vi "Close.vi"(8 "error in":errorcluster, 11 "OnOff in":refnum<class "OnOff.lvclass">) -> (0 "error out":errorcluster, 3 "OnOff out":refnum<class "OnOff.lvclass">)   [LabVIEW 2023, in "OnOff.lvclass"]
uses:
  OnOff.lvclass
  OnOff.lvclass/OnOff.ctl
  <vilib>/ADAS Replay HIL/AdasHilServices/AdasHilServices Fill In Error Info Ex.vi
  <vilib>/ADAS Replay HIL/AdasHilServices/AdasHilChannelServices.lvlib
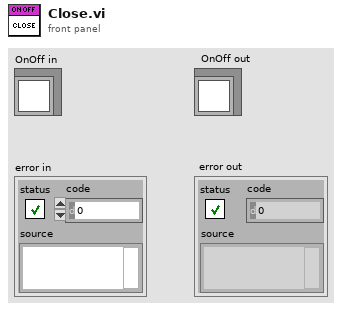
[diagram p1: front panel]
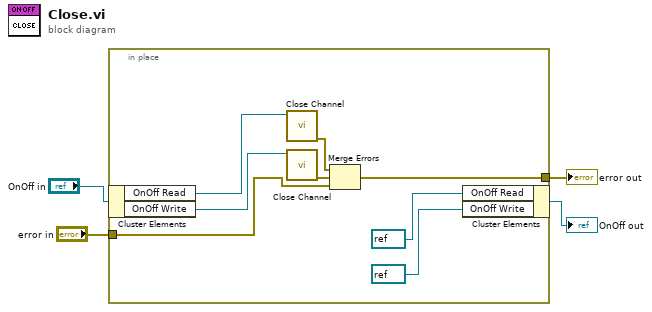
[diagram p0: block diagram]
diagram:
  n1 = in-place {
    in-place-border: "error in" -> [w12]
    in-place-border: [w11] -> w2
    n2 = in-place-cluster #1("OnOff in") -> ("OnOff Read"=w10:refnum<k21>, "OnOff Write"=w9:refnum<k21>)
    n3 = call <vilib>:"Close Channel.vi"("ADAS HIL Channel"=w10) -> ("error out"=w6:errorcluster)  [unwired: 10 in]
    n4 = call <vilib>:"Close Channel.vi"("ADAS HIL Channel"=w9) -> ("error out"=w5:errorcluster)  [unwired: 10 in]
    n5 = Merge Errors(w6, w5, w12) -> (w11:errorcluster)
    n6 = in-place-cluster #1("OnOff Read"=refnum<k21> refnum, "OnOff Write"=refnum<k21> refnum) -> (→"OnOff out":refnum<class "OnOff.lvclass">)
  }
  "error out" <- w2
